vi "SigGen-Compute Max Level (arbitrary).vi"(0 "Stimulus Channel":T22(xcontrol), 5 "Y":dbl[](array[numeric]), 7 "Sampling Rate (Hz)":dbl, 9 "Npts":i32, 11 "error in (no error)":errorcluster) -> (4 "Stimulus Channel out":T22(xcontrol), 14 "Max Level":dbl, 15 "error out":errorcluster)   [LabVIEW 2020]
uses:
  Controls/Stimulus Channel XCtl/Stimulus Channel.xctl
  PXI DAQ VIs/DAQ Engine VIs/PXI Globals.vi
  Utility VIs/Math VIs/Linear to dB (scalar).vi
  Utility VIs/Math VIs/FFT x(t) to dB,Degrees (1D).vi
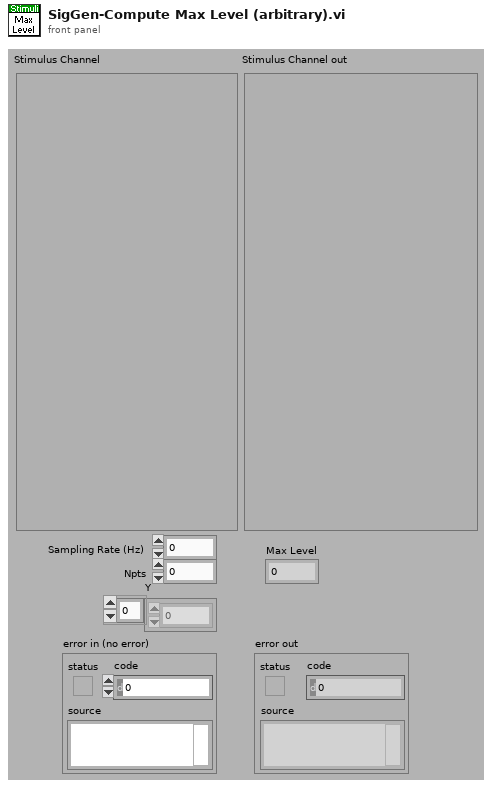
[diagram p1: front panel]
types:
  T1 = typedef "Waveform XCtl.xctl/Waveform Data.ctl" = cluster{"Type":T2, "Tone":T3, "Pulse Train":T4, "Noise":T7, "File":T8, "FMSweep":T9, "Chirp Train":T10, "Complex Tone":cluster{"Params":T12, "Data":T14}, "Moving Ripple":T15}
  T2 = typedef "Waveform Enum.ctl" = enum16{"OFF", "Tone", "Noise", "Pulse Train", "File", "FM Sweep", "Chirp Train", "Complex Tone", "FM Tone", "Moving Ripple"}
  T3 = typedef "Tone Params.ctl" = cluster{"Frequency (kHz)":dbl, "Last Freq":dbl, "Last Phase":dbl}
  T4 = typedef "Pulse Train Params.ctl" = cluster{"Pulse width (us)":dbl, "Pulse rate (Hz)":dbl, "Gap (ms)":dbl, "Polarity":T5, "PT State":T6, "Asynch":bool}
  T5 = typedef "Pulse Polarity.ctl" = enum16{"POS", "NEG", "POS-NEG", "NEG-POS"}
  T6 = typedef "PT-Continuous State.ctl" = cluster{"Template":dbl[], "Nperiod":i32, "Index":i32, "Pulse Rate (Hz)":dbl, "Phase (cycles)":dbl, "Noff":i32}
  T7 = typedef "Noise Params.ctl" = cluster{"InvFilt":bool, "Noise":dbl[], "CurPt":i32, "Aweight":bool, "Seed":i32, "afile":path}
  T8 = typedef "StimFile-Params.ctl" = cluster{"Filename":path, "Signal":dbl[], "Channel":i32, "stream":bool, "offset":i32, "nreps":i32, "loops":i32, "Randomize":bool, "order":i32[], "Seed":i32, "Tokens":i32}
  T9 = typedef "FM Sweep Params.ctl" = cluster{"Rate (oct/s)":dbl, "Fmin (Hz)":dbl, "Fmax (Hz)":dbl, "Ramp (ms)":dbl, "Linear":bool}
  T10 = typedef "Chirp Train.ctl" = cluster{"Params":T11, "Data":cluster{"WF":dbl[]}}
  T11 = typedef "Chirp Train Params.ctl" = cluster{"Fmin (kHz)":dbl, "Fmax (kHz)":dbl, "Compensate":bool, "Duration (ms)":dbl}
  T12 = typedef "CT-Params.ctl" = cluster{"F0 (Hz)":dbl, "Band":cluster{"Flow (Hz)":dbl, "Fhigh (Hz)":dbl}, "Phase":T13, "Min F0 (Hz)":dbl, "Max F0 (Hz)":dbl, "ContinRandPhase":bool, "Max peak factor":dbl, "Max mod depth":dbl, "MinHarmNum":i32, "MaxHarmNum":i32, "Level Mode":enum16{"per component", "overall rms"}, "% jitter":dbl}
  T13 = typedef "CT-Phase Enum.ctl" = enum16{"Cosine", "Random", "Alternating"}
  T14 = typedef "CT-Runtime Data.ctl" = cluster{"Ncomp":i32, "MinHarm":i32, "Phase":dbl[], "Amplitude":dbl[], "Npts/frame":i32, "Last F0":dbl, "Fmin":dbl, "Fmax":dbl, "Lslope":dbl, "randphase":bool, "overall rms":bool, "fmult":dbl[], "jittered":bool}
  T15 = typedef "Moving Ripple.ctl" = cluster{"Params":T16, "Data":T17}
  T16 = typedef "Moving Ripple.Params.ctl" = cluster{"Fmin":dbl, "Fmax":dbl, "Density":dbl, "Velocity":dbl, "Depth":dbl, "Phase":dbl, "Comp/oct":i32}
  T17 = typedef "Moving Ripple.Data.ctl" = cluster{"Freq":dbl[], "A":dbl[], "phase":dbl[], "Phase":dbl}
  T18 = typedef "Filter XCtl.xctl/Filter Data.ctl" = cluster{"CF (kHz)":dbl, "BW (kHz)":dbl, "IIR Filter Cluster":cluster{"filter structure":enum32{"IIR 2nd Order", "IIR 4th Order"}, "Reverse Coefficients":dbl[], "Forward Coefficients":dbl[]}, "Final Filter State":dbl[], "Scale Factor":dbl, "Final Filter State 2":dbl[], "Quadrature":bool, "Type":enum16{"Lowpass", "Highpass", "Bandpass", "Bandstop", "OFF"}}
  T19 = typedef "Gate Control.xctl/Gate Data.ctl" = cluster{"Active":bool, "Delay (ms)":dbl, "Width (ms)":dbl, "Ramp (ms)":dbl}
  T20 = typedef "Level XCtl.xctl/Level Data.ctl" = cluster{"Level":dbl, "Units":T21, "Max":dbl, "Multiplier":dbl, "Cal File":path, "Cal":cluster{"Freq (Hz)":dbl[], "Mag (dB SPL)":dbl[], "Phase (deg)":dbl[]}}
  T21 = typedef "Level Units.ctl" = enum16{"dB atten", "dB SPL", "dB re 1 Vrms", "dB V/Hz½", "mW", "dB HL", "Volts", "dB mW"}
  T22 = cluster{"Waveform":T1, "Filter":T18, "Gate":T19, "Level":T20}
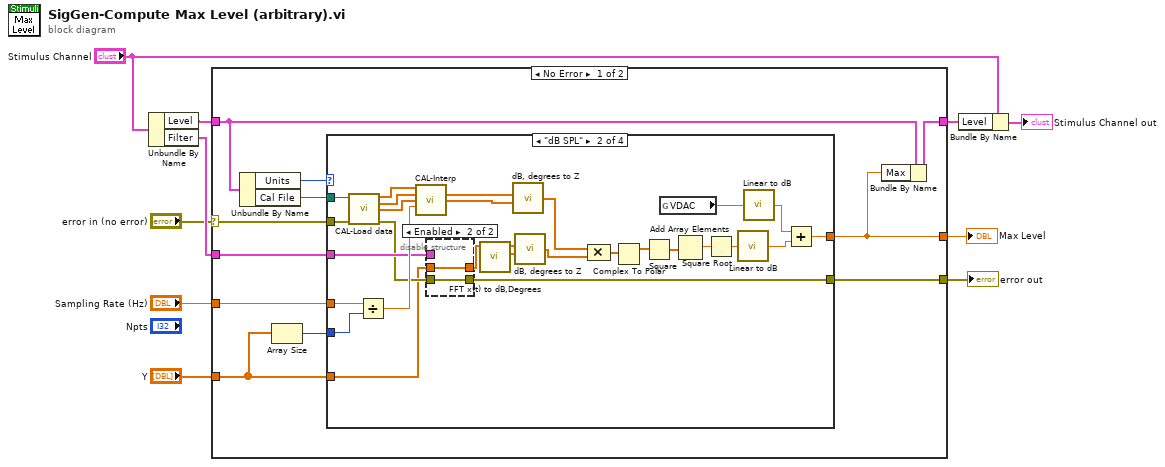
[diagram p0: block diagram]
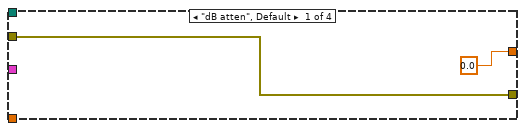
[diagram p2: hidden frame]
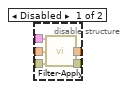
[diagram p3: hidden frame]
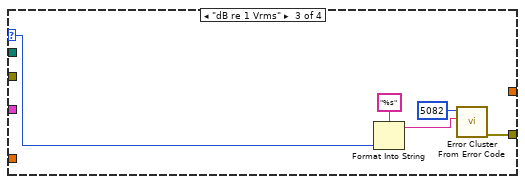
[diagram p4: hidden frame]
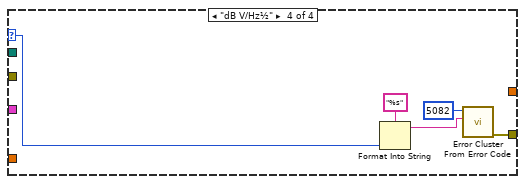
[diagram p5: hidden frame]
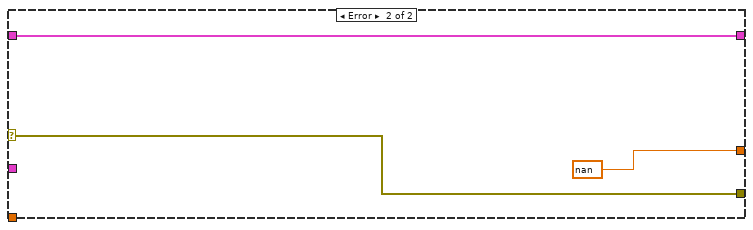
[diagram p6: hidden frame]
diagram:
  n1 = Unbundle By Name("Stimulus Channel") -> ("Level"=w8:T20, "Filter"=w6:T18)
  n2 = case shown="No Error" "error in (no error)" {
    selector: "error in (no error)" -> [w21 w71]
    tunnel: w8 -> [w18 w69]
    tunnel: w6 -> [w20 _]
    tunnel: [w19 w71] -> w4
    tunnel: [w17 nan ("Reference Level")] -> w7
    tunnel: [w16 w69] -> w3
    tunnel: "Y" -> [w12 _]
    tunnel: "Sampling Rate (Hz)" -> [w13 _]
    frame No Error {
      n3 = Unbundle By Name(w18) -> ("Units"=w15:T21, "Cal File"=w14:path)
      n4 = Array Size(array=w12) -> (size(s)=w11:i32)
      n5 = case shown="\"dB SPL\"" w15 {
        selector: w15 -> [_ _ w60 w64]
        tunnel: w21 -> [w22 w51 _ _]
        tunnel: w20 -> [_ w29 _ _]
        tunnel: [0.0 ("Reference Level") w49 _ _] -> w17
        tunnel: [w22 w27 w63 w65] -> w19
        tunnel: w14 -> [_ w47 _ _]
        tunnel: w12 -> [_ w26 _ _]
        tunnel: w13 -> [_ w37 _ _]
        tunnel: w11 -> [_ w38 _ _]
        frame "dB atten", Default {
        }
        frame "dB SPL" {
          n6 = call "CAL-Load data.vi"("user path"=w47, "error in (no error)"=w51) -> ("Frequency (Hz)"=w44:dbl[], "Mag"=w43:dbl[], "Phase"=w42:dbl[], "error out"=w28:errorcluster)  [unwired: 6 in, 4 out]
          n7 = Divide(x=w37, y=w38) -> (x/y=w39:dbl)
          n8 = call "CAL-Interp.vi"("Frequency (Hz)"=w44, "Magnitude (dB)"=w43, "Phase (degrees)"=w42, "df (Hz)"=w39) -> ("Interp Magnitude (dB)"=w41:dbl[], "Interp Phase (degrees)"=w40:dbl[])  [unwired: 8 in, 2 out]
          n9 = disable-structure shown="Enabled" {
            disable-tunnel: w29 -> [w56 _]
            disable-tunnel: w28 -> [w55 w57]
            disable-tunnel: [w54 w57] -> w27
            disable-tunnel: w26 -> [w53 w58]
            disable-tunnel: [w52 w58] -> w25
            frame Disabled {
              n10 = call "Filter-Apply.vi"("Filter"=w56, "X"=w53, "error in (no error)"=w55) -> ("Filtered X"=w52:dbl[], "error out"=w54:errorcluster)  [unwired: 10 in, 1 out]
            }
            frame Enabled {
            }
          }
          n11 = call-poly "FFT x(t) to dB,Degrees.vi"("X"=w25) -> ("+Freq Phase of FFT (degrees)"=w35:dbl[], "+Freq. Mag of FFT (dB rms)"=w36:dbl[])  [unwired: 8 in, 1 out]
          n12 = call "dB, degrees to Z.vi"("Magnitude (dB)"=w41, "Phase (degrees)"=w40) -> ("Z"=w45:cdb[])  [unwired: 5 in]
          n13 = call "dB, degrees to Z.vi"("Magnitude (dB)"=w36, "Phase (degrees)"=w35) -> ("Z"=w24:cdb[])  [unwired: 5 in]
          n14 = Compound Arithmetic op=MULTIPLY(w45, w24) -> (w46:cdb[])
          n15 = Complex To Polar(r * e^(i*theta)=w46) -> (r=w31:dbl[])  [unwired: 1 out]
          n16 = Square(x=w31) -> (x^2=w34:dbl[])
          n17 = global read "PXI Globals.vi" "VDAC"() -> (w50:dbl)
          n18 = Add Array Elements(numeric array=w34) -> (sum=w33:dbl)
          n19 = Square Root(x=w33) -> (sqrt(x)=w32:dbl)
          n20 = call-poly "Linear to dB.vi"("Linear"=w32) -> ("dB"=w30:dbl)
          n21 = call-poly "Linear to dB.vi"("Linear"=w50) -> ("dB"=w48:dbl)
          n22 = Add(x=w48, y=w30) -> (x+y=w49:dbl)
        }
        frame "dB re 1 Vrms" {
          n23 = Format Into String(format string="%s", w60) -> (resulting string=w61:string)  [unwired: 2 in, 1 out]
          n24 = call <vilib>:"Error Cluster From Error Code.vi"("error message (\"\")"=w61, "error code (0)"=5082) -> ("error out"=w63:errorcluster)  [unwired: 7 in]
        }
        frame "dB V/Hz½" {
          n25 = Format Into String(format string="%s", w64) -> (resulting string=w67:string)  [unwired: 2 in, 1 out]
          n26 = call <vilib>:"Error Cluster From Error Code.vi"("error message (\"\")"=w67, "error code (0)"=5082) -> ("error out"=w65:errorcluster)  [unwired: 7 in]
        }
      }
      n27 = Bundle By Name(cluster=w18, "Max"=w17) -> (w16:T20)
    }
    frame Error {
    }
  }
  "error out" <- w4
  "Max Level" <- w7
  n28 = Bundle By Name(cluster="Stimulus Channel", "Level"=w3) -> (→"Stimulus Channel out":T22)
